vi "LVObject to JSON - Error Serialization Binder - Returns Error.vi"() -> ()   [LabVIEW 2017, in "Generic Object Serializer Tests.lvlib" / "Serialization Binder.lvlib"]
uses:
  Serialization Binder.lvlib
  Generic Object Serializer/Generic Object Serializer.lvclass
  Error Serialization Binder/Error Serialization Binder.lvclass
  C:/Users/de200256/Code/logmanoriginal/jsontext-object-serialization/Serialization Binder/Serialization Binder.lvclass
  Generic Object Serializer/Type Name Handling.ctl
  Generic Object Serializer/Generic Object Serializer.lvclass/Generic Object Serializer.ctl
  Generic Object Serializer/Write Serialization Binder.vi
  Generic Object Serializer/Write Type Name Handling.vi
  <vilib>/addons/_JKI Toolkits/Caraya/classes/Test/Test.lvclass
  <vilib>/addons/_JKI Toolkits/Caraya/classes/Assert/Assert.lvclass
panel:
  out "error out":errorcluster
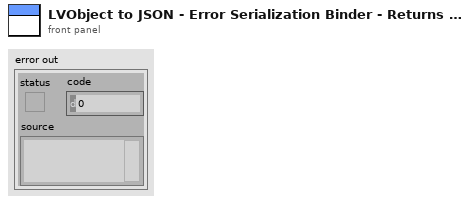
[diagram p1: front panel]
types:
  T1 = typedef "Generic Object Serializer.lvclass/Type Name Handling.ctl" = enum16{"None", "Inline"}
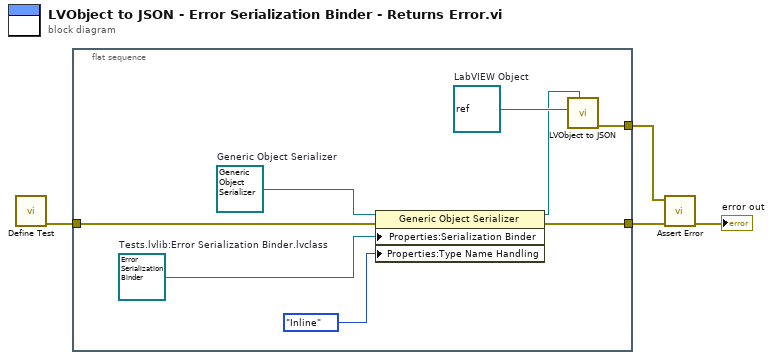
[diagram p0: block diagram]
diagram:
  n1 = call <vilib>:"Define Test.vi"() -> ("error out"=w4:errorcluster)  [unwired: 11 in]
  n2 = flat-sequence {
    tunnel: [w7] -> w3
    tunnel: w4 -> [w11]
    tunnel: [w6] -> w1
    frame #0 {
      w9 = refnum<class> refnum  # LabVIEW Object
      w10 = refnum<class "Error Serialization Binder.lvclass"> refnum  # Tests.lvlib:Error Serialization Binder.lvclass
      w12 = refnum<class "Generic Object Serializer.lvclass"> refnum  # Generic Object Serializer
      n3 = property class="Generic Object Serializer"(reference=w12, error in=w11, "Properties:Serialization Binder"=w10, "Properties:Type Name Handling"=Type_Name_Handling."Inline" ("Type Name Handling")) -> (reference out=w8:refnum<class "Generic Object Serializer.lvclass">, error out=w7:errorcluster)
      n4 = call-dynamic "LVObject to JSON.vi"("LVClass Serializer"=w8, "Object"=w9) -> ("error out"=w6:errorcluster)  [unwired: 8 in, 1 out]
    }
  }
  n5 = call <vilib>:"Assert Error.vi"("error in (no error)"=w3, "Error?"=w1) -> ("error out"=→"error out":errorcluster)  [unwired: 9 in]
